vi "IPC-Modbus-U8ArrayToBitArray.vi"(8 "U8 Array":u8[](array[numeric]), 9 "Bit Array size":u16) -> (3 "Bit Array":bool[](array[boolean]))   [LabVIEW 2014]
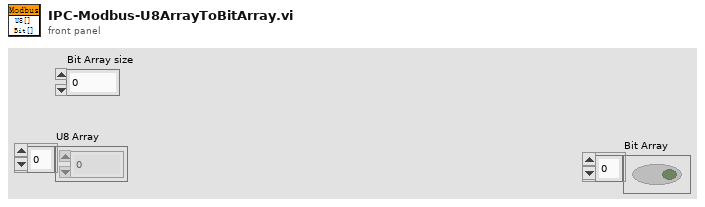
[diagram p1: front panel]
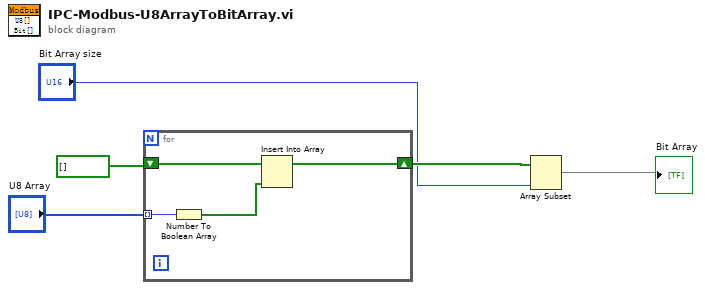
[diagram p0: block diagram]
diagram:
  n1 = for {
    tunnel: "U8 Array" -> [w9] mode=indexing
    shift-right: [w6] -> w3
    shift-left: bool[] [] -> [w7]
    n2 = Number To Boolean Array(number=w9) -> (Boolean array=w8:bool[])
    n3 = Insert Into Array(array=w7, new element=w8) -> (w6:bool[])  [unwired: 1 in]
  }
  n4 = Array Subset(array=w3, length="Bit Array size") -> (→"Bit Array":bool[])  [unwired: 1 in]
